vi "stop_stimulation.vi"(8 "error in (no error)":errorcluster, 11 "DL090503StimulatorScaffold in":refnum<class "StimulatorDL090503.lvclass">) -> (0 "error out":errorcluster, 3 "DL090503StimulatorScaffold out":refnum<class "StimulatorDL090503.lvclass">)   [LabVIEW 2010, in "StimulatorDL090503.lvclass"]
uses:
  StimulatorDL090503.lvclass
  StimulatorDL090503.lvclass/StimulatorDL090503.ctl
  SignalWriter/GenericSignalWriter/GenericSignalWriter/GenericSignalWriter.lvclass
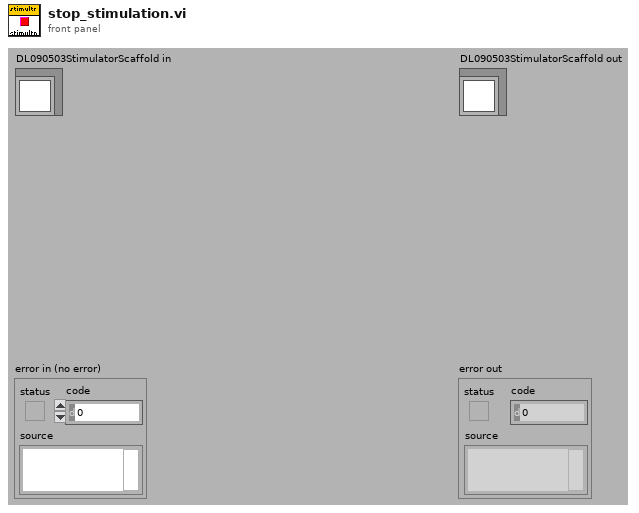
[diagram p1: front panel]
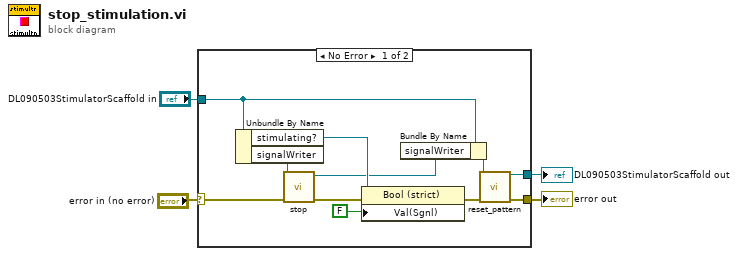
[diagram p0: block diagram]
diagram:
  n1 = case shown="No Error" "error in (no error)" {
    selector: "error in (no error)" -> [w12 w17]
    tunnel: [w6 w17] -> w4
    tunnel: [w5 w16] -> w3
    tunnel: "DL090503StimulatorScaffold in" -> [w10 w16]
    frame No Error {
      n2 = Unbundle By Name(w10) -> ("stimulating?"=w14:refnum<vi>, "signalWriter"=w13:refnum<class "GenericSignalWriter.lvclass">)
      n3 = call-dynamic "stop.vi"("error in (no error)"=w12, "WriteSignalsGenericPlugin in"=w13) -> ("error out"=w11:errorcluster, "WriteSignalsGenericPlugin out"=w9:refnum<class "GenericSignalWriter.lvclass">)  [unwired: 8 out]
      n4 = property class="Bool (strict)"(reference=w14, error in=w11, "Val(Sgnl)"=FALSE ("Value (Signaling)")) -> (error out=w8:errorcluster)  [unwired: 1 out]
      n5 = Bundle By Name(cluster=w10, "signalWriter"=w9) -> (w7:refnum<class "StimulatorDL090503.lvclass">)
      n6 = call "reset_pattern.vi"("error in (no error)"=w8, "StimulatorDL090503 in"=w7) -> ("error out"=w6:errorcluster, "StimulatorDL090503 out"=w5:refnum<class "StimulatorDL090503.lvclass">)  [unwired: 8 in]
    }
    frame Error {
    }
  }
  "error out" <- w4
  "DL090503StimulatorScaffold out" <- w3
